vi "Write DO Lines.vi"(8 "error in (no error)":errorcluster, 10 "DO Lines":bool[](array[boolean]), 11 "Set Output Lines Msg in":refnum<class "Set Output Lines Msg.lvclass">) -> (0 "error out":errorcluster, 3 "Set Output Lines Msg out":refnum<class "Set Output Lines Msg.lvclass">)   [LabVIEW 2021, in "BNT_ULx.lvlib" / "Set Output Lines Msg.lvclass"]
uses:
  Set Output Lines Msg.lvclass
  Set Output Lines Msg.lvclass/Set Output Lines Msg.ctl
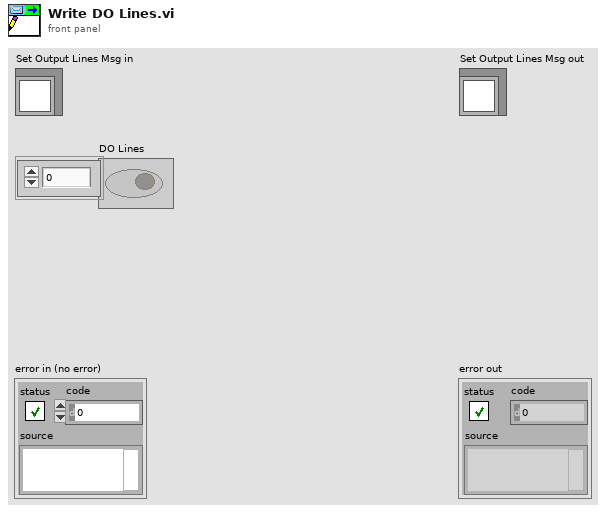
[diagram p1: front panel]
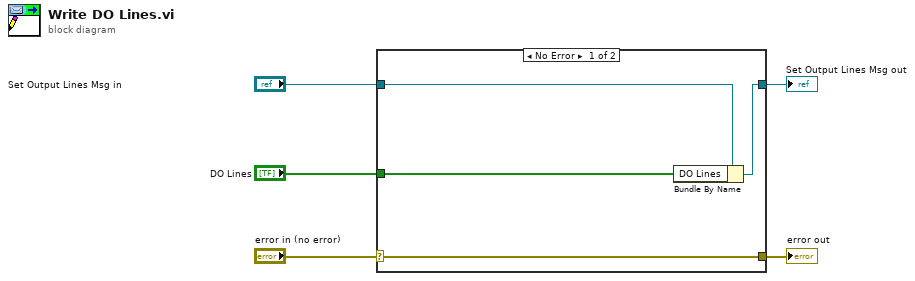
[diagram p0: block diagram]
diagram:
  n1 = case shown="No Error" "error in (no error)" {
    selector: "error in (no error)" -> [w9 w10]
    tunnel: [w9 w10] -> w4
    tunnel: [w7 w11] -> w2
    tunnel: "Set Output Lines Msg in" -> [w8 w11]
    tunnel: "DO Lines" -> [w6 _]
    frame No Error {
      n2 = Bundle By Name(cluster=w8, "DO Lines"=w6) -> (w7:refnum<class "Set Output Lines Msg.lvclass">)
    }
    frame Error {
    }
  }
  "error out" <- w4
  "Set Output Lines Msg out" <- w2
